vi "Unit conversion.vi"(8 "Value to convert":dbl format="%#_13g", 9 "Ending Units":u16(ring) items=["Wavenumber (cm-1)", "Frequency (THz)", "Wavelength (nm)"], 10 "Starting Units":u16(ring) items=["Wavenumber (cm-1)", "Frequency (THz)", "Wavelength (nm)"]) -> (0 "Output":dbl format="%#_19g")   [LabVIEW 2017]
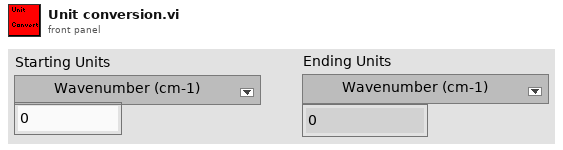
[diagram p1: front panel]
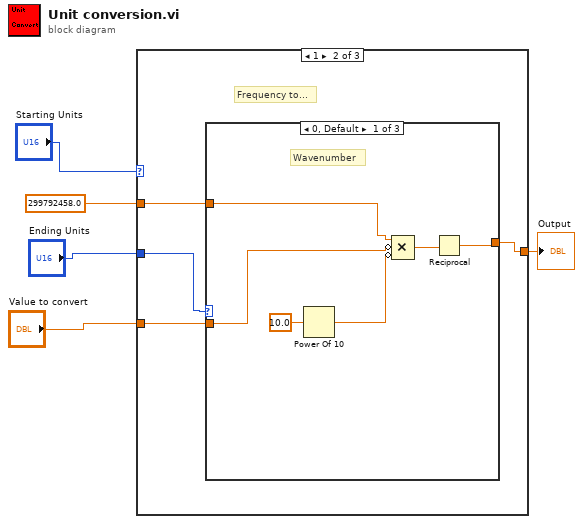
[diagram p0: block diagram]
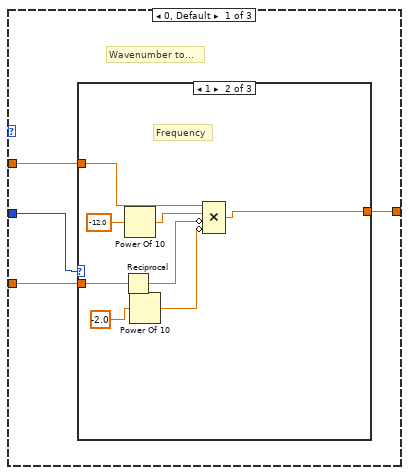
[diagram p2: hidden frame]
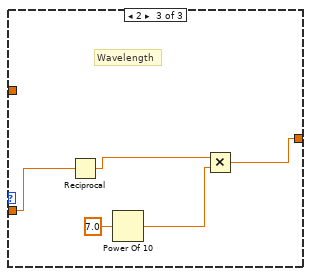
[diagram p4: hidden frame]
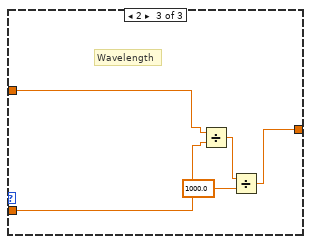
[diagram p6: hidden frame]
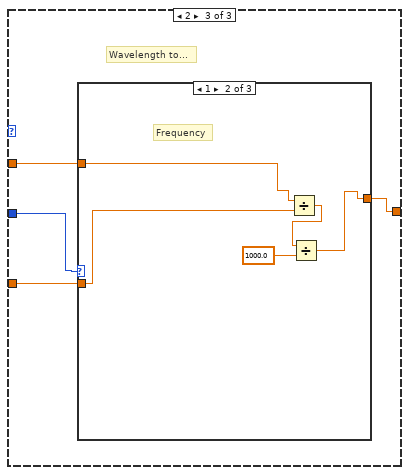
[diagram p7: hidden frame]
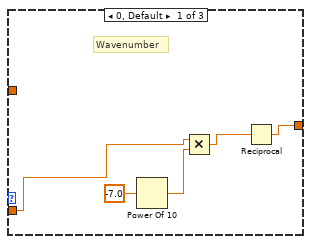
[diagram p8: hidden frame]
diagram:
  n1 = case shown="1" "Starting Units" {
    tunnel: "Ending Units" -> [w9 w27 w43]
    tunnel: 299792458.0 -> [w8 w24 w40]
    tunnel: "Value to convert" -> [w7 w26 w41]
    tunnel: [w6 w25 w42] -> w1
    frame 0, Default {
      # "Wavenumber to..."
      n2 = case shown="1" w9 {
        tunnel: w8 -> [_ w16 _]
        tunnel: w7 -> [w10 w18 w23]
        tunnel: [w10 w11 w22] -> w6
        frame 0, Default {
          # "Wavenumber"
        }
        frame 1 {
          # "Frequency"
          n3 = Reciprocal(x=w18) -> (1/x=w14:dbl)
          n4 = Power Of 10(x=-12.0) -> (10^x=w12:dbl)
          n5 = Power Of 10(x=-2.0) -> (10^x=w15:dbl)
          n6 = Compound Arithmetic op=MULTIPLY(w16, w12, invert w14, invert w15) -> (w11:dbl)
        }
        frame 2 {
          # "Wavelength"
          n7 = Reciprocal(x=w23) -> (1/x=w20:dbl)
          n8 = Power Of 10(x=7.0) -> (10^x=w21:dbl)
          n9 = Multiply(x=w20, y=w21) -> (x*y=w22:dbl)
        }
      }
    }
    frame 1 {
      # "Frequency to..."
      n10 = case shown="0, Default" w27 {
        tunnel: w26 -> [w30 w34 w38]
        tunnel: [w33 w34 w35] -> w25
        tunnel: w24 -> [w31 _ w39]
        frame 0, Default {
          # "Wavenumber"
          n11 = Power Of 10(x=10.0) -> (10^x=w28:dbl)
          n12 = Compound Arithmetic op=MULTIPLY(w31, invert w30, invert w28) -> (w32:dbl)
          n13 = Reciprocal(x=w32) -> (1/x=w33:dbl)
        }
        frame 1 {
          # "Frequency"
        }
        frame 2 {
          # "Wavelength"
          n14 = Divide(x=w39, y=w38) -> (x/y=w36:dbl)
          n15 = Divide(x=w36, y=1000.0) -> (x/y=w35:dbl)
        }
      }
    }
    frame 2 {
      # "Wavelength to..."
      n16 = case shown="1" w43 {
        tunnel: [w48 w49 w54] -> w42
        tunnel: w41 -> [w44 w52 w54]
        tunnel: w40 -> [_ w53 _]
        frame 0, Default {
          # "Wavenumber"
          n17 = Power Of 10(x=-7.0) -> (10^x=w45:dbl)
          n18 = Multiply(x=w44, y=w45) -> (x*y=w46:dbl)
          n19 = Reciprocal(x=w46) -> (1/x=w48:dbl)
        }
        frame 1 {
          # "Frequency"
          n20 = Divide(x=w53, y=w52) -> (x/y=w50:dbl)
          n21 = Divide(x=w50, y=1000.0) -> (x/y=w49:dbl)
        }
        frame 2 {
          # "Wavelength"
        }
      }
    }
  }
  "Output" <- w1
